vi "everything.vi"() -> ()   [LabVIEW 2019]
uses:
  <vilib>/Instr/_visa.llb/VISA Set IO Buffer Mask.ctl
  <vilib>/Instr/_visa.llb/VISA Configure Serial Port (Instr).vi
  <vilib>/express/express shared/transition.llb/Dynamic To Waveform Array.vi
  <vilib>/express/express arith-compare/Formula/Block/exnFormulaBlock how many pts in the wave.vi
  <vilib>/express/express shared/ex_Modify Signal Name.vi
  <vilib>/express/express shared/transition.llb/Waveform Array To Dynamic.vi
  <vilib>/express/express arith-compare/Formula/XNode/ExpressFormulaBlockNode.xnode
panel:
  out "VI Name":string
  out "Voltage 3":dbl format="%.2g"
  out "CFM 3":dbl format="%.2g"
  out "Average CFM 3":dbl format="%.1g"
  out "Voltage 2":dbl format="%#.2g"
  out "CFM 2":dbl format="%.2g"
  out "Average CFM 2":dbl format="%.1g"
  out "CFM 1":dbl format="%.2g"
  out "Average CFM 1":dbl format="%.1g"
  out "Voltage 1":dbl format="%#.2g"
  in  "% Power":dbl min=0.0 max=100.0 step=1.0
  out "Required Voltage":dbl
  out "main return":dbl
  out "t4":dbl
  out "zone 2":dbl
  out "t3":dbl
  out "outlet":dbl
  out "t6":dbl
  out "zone 1":dbl
  out "t5":dbl
  out "t2":dbl
  out "h2":dbl
  out "t1":dbl
  out "h3":dbl
  out "inlet air":dbl
  out "h4":dbl
  out "h1":dbl
  out "h6":dbl
  out "zone 3":dbl
  out "h5":dbl
  in  "Stop":bool
  in  "zone 1 inlet":dbl min=0.0 max=100.0
  in  "zone 1 return":dbl min=0.0 max=100.0
  in  "Fans":i32 min=0 max=1
  in  "zone 2 inlet":dbl min=0.0 max=100.0
  in  "zone 3 inlet":dbl min=0.0 max=100.0
  in  "zone 2 return":dbl min=0.0 max=100.0
  in  "zone 1 co2":dbl min=0.0 max=100.0
  in  "Light 1":i32 min=0 max=1
  in  "fresh air":dbl min=0.0 max=100.0
  in  "zone 2 co2":dbl min=0.0 max=100.0
  in  "Light 3":i32 min=0 max=1
  in  "zone 3 return":dbl min=0.0 max=100.0
  in  "Light 2":i32 min=0 max=1
  in  "zone 3 co2":dbl min=0.0 max=100.0
  in  "VISA- Arduino Uno":refnum<visa-resource-name>
  in  "VISA- Arduino Mega":refnum<visa-resource-name>
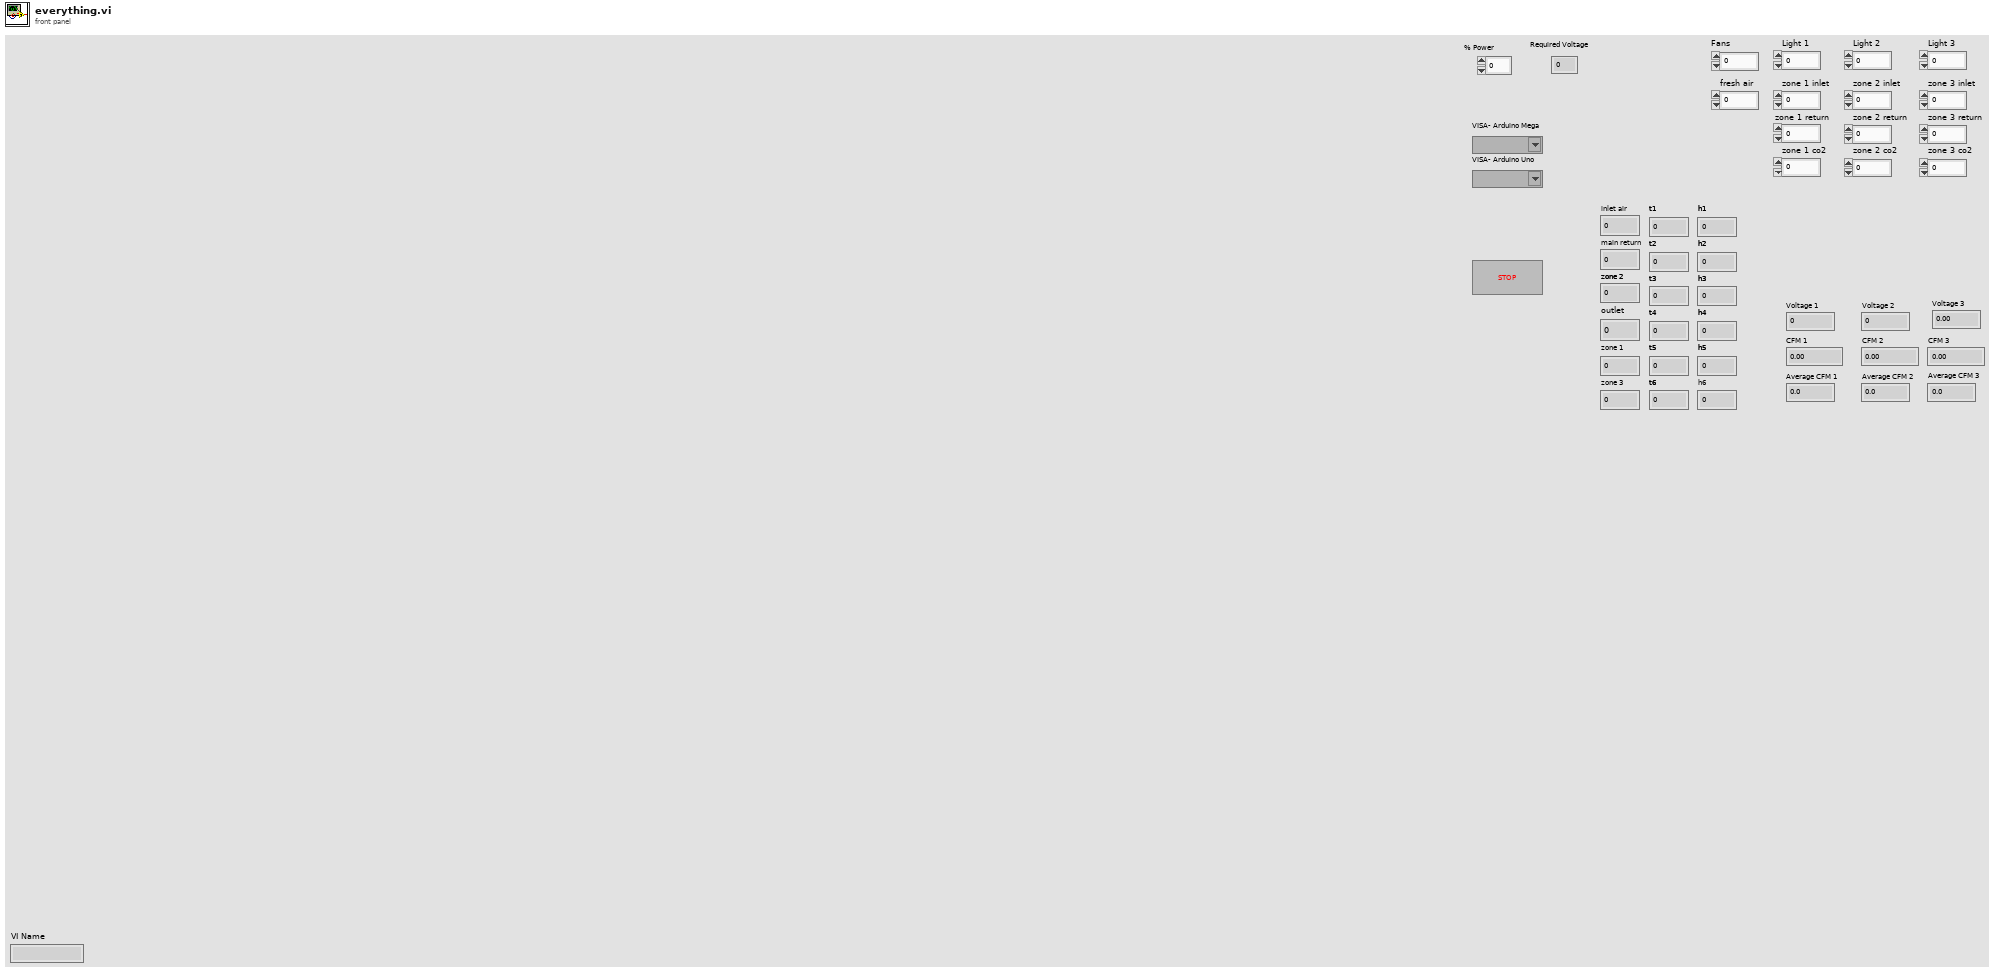
[diagram p1: front panel]
types:
  T1 = typedef "VISA Set IO Buffer Mask.ctl" = u16
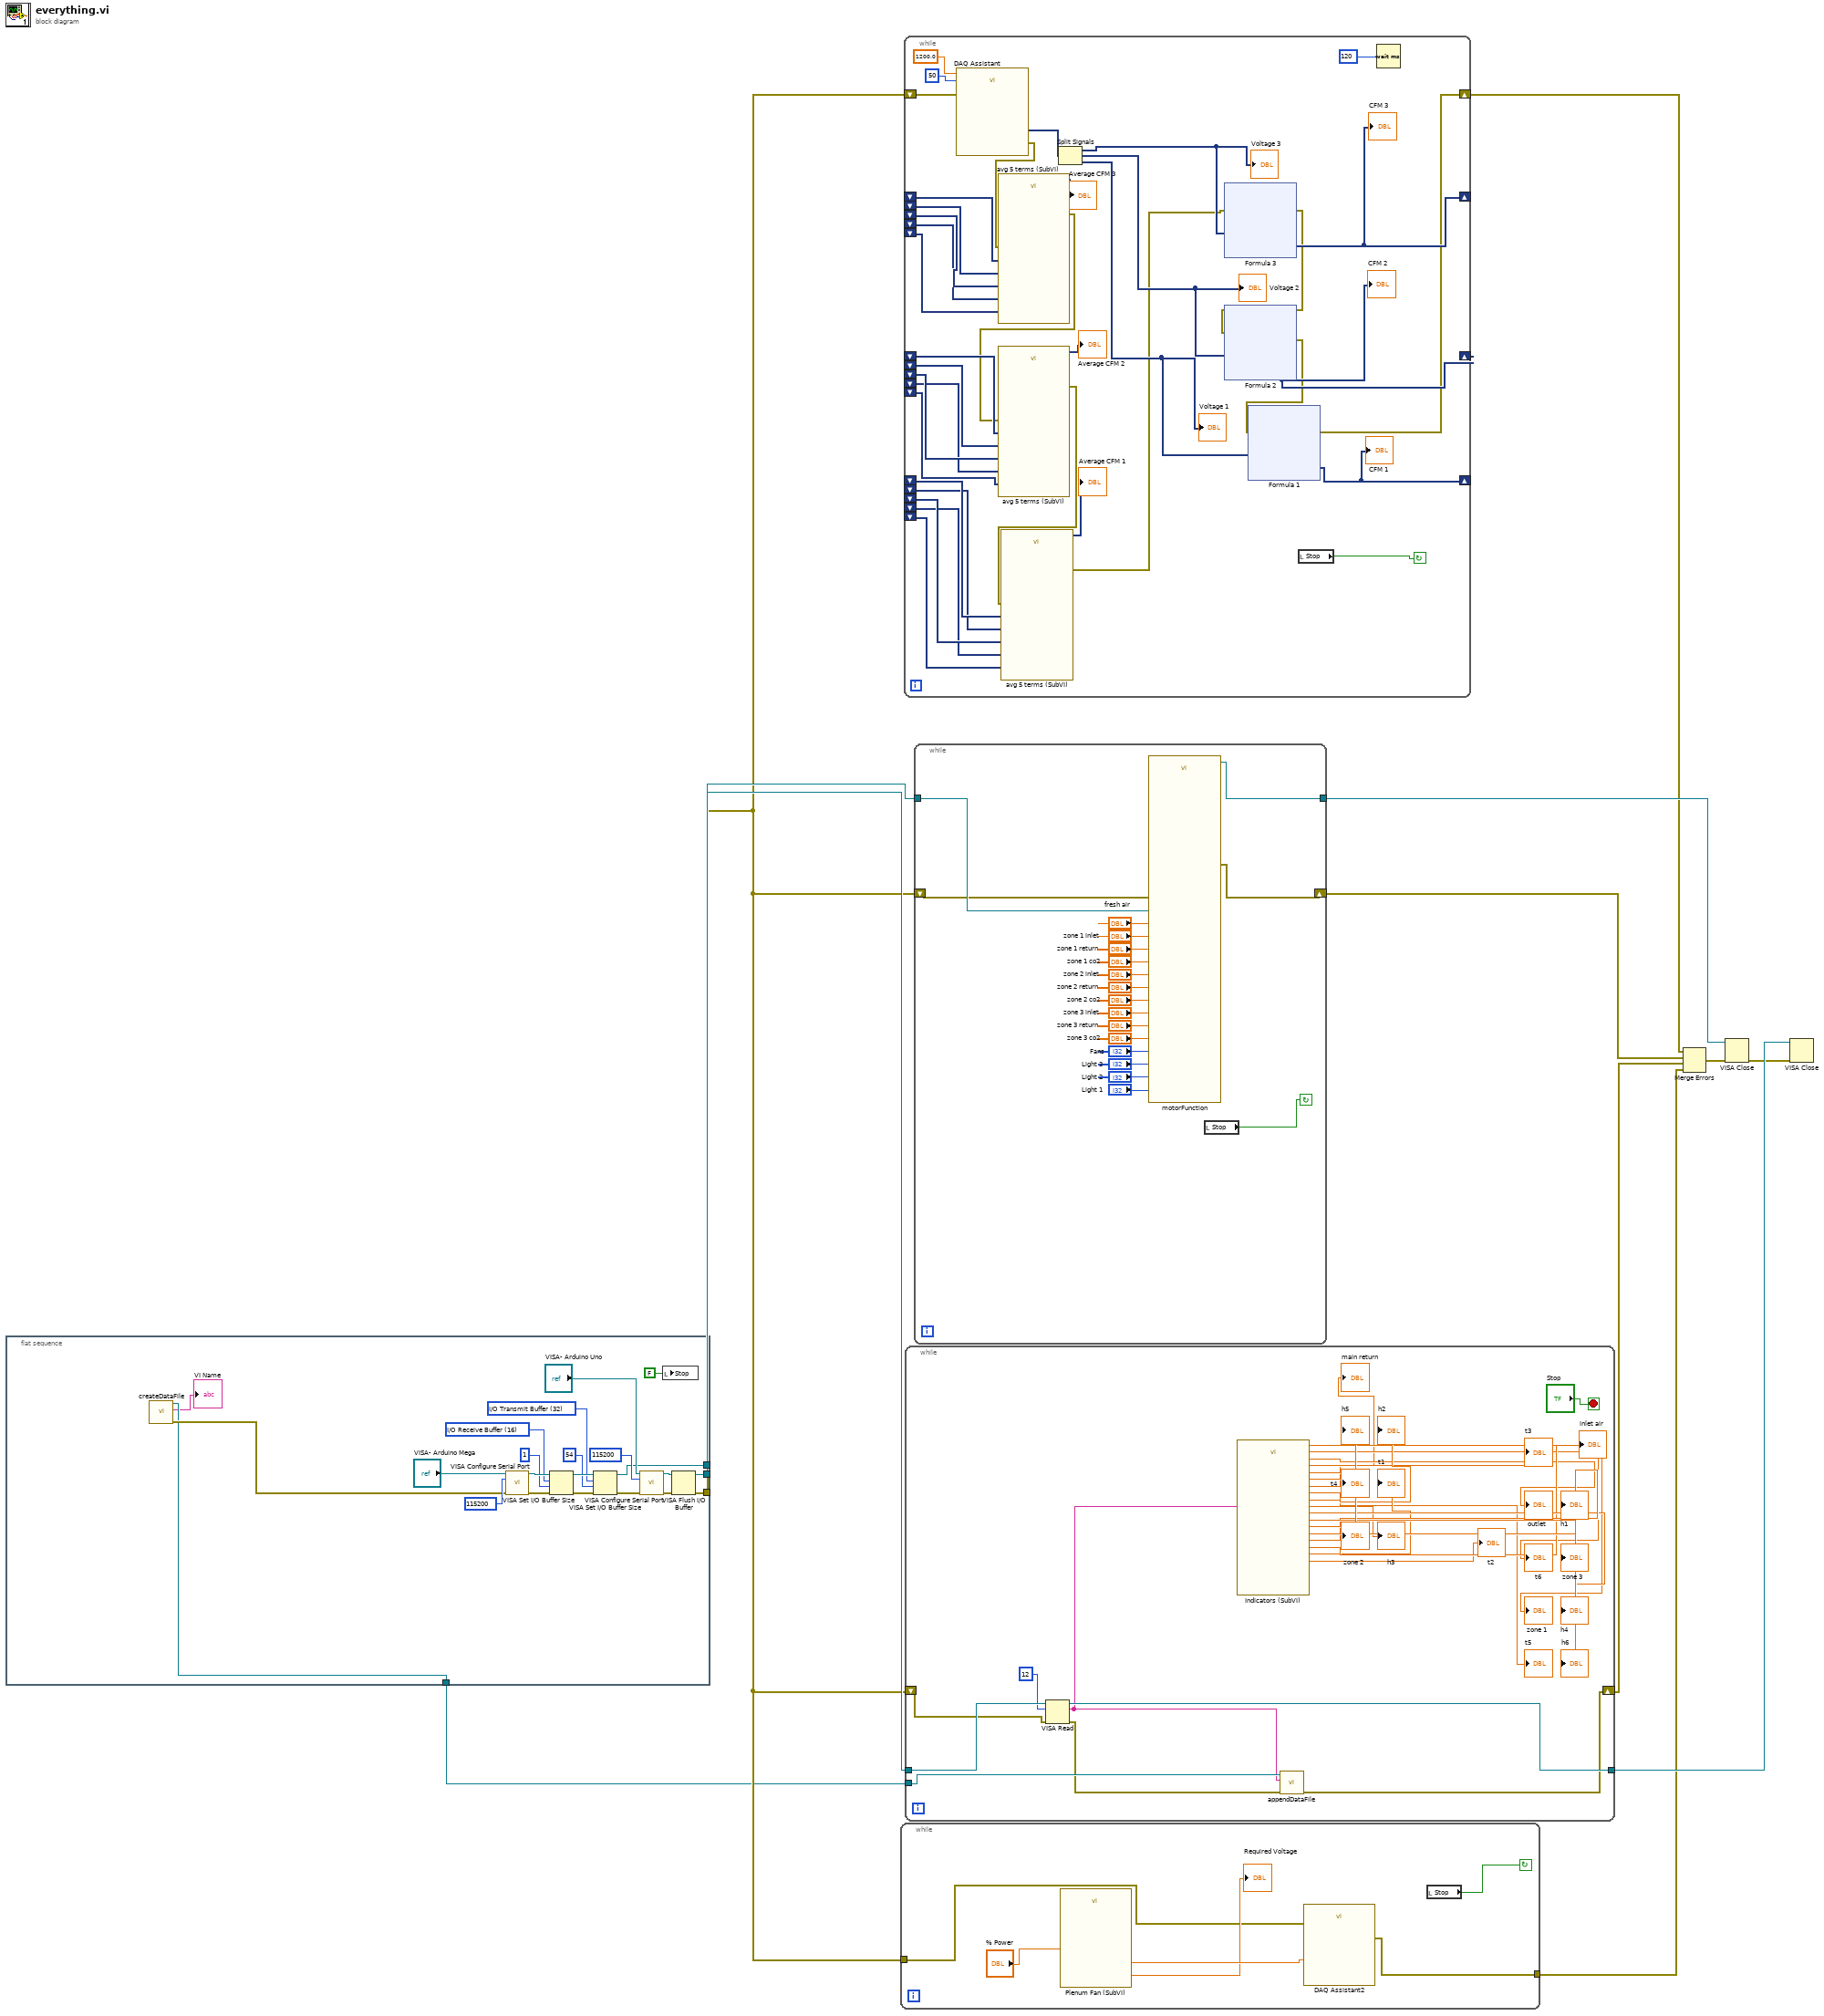
[diagram p0: block diagram]
diagram:
  n1 = flat-sequence {
    tunnel: [w20] -> w12
    tunnel: [w19] -> w11
    tunnel: [w17] -> w3
    tunnel: [w14] -> w1
    frame #0 {
      w27 = T1 32 items=["I/O Receive Buffer"=16, "I/O Transmit Buffer"=32, "I/O Receive and Transmit Buffer"=48] ("Mask")
      w30 = T1 16 items=["I/O Receive Buffer"=16, "I/O Transmit Buffer"=32, "I/O Receive and Transmit Buffer"=48] ("Mask")
      n2 = call "createDataFile.vi"() -> ("error out"=w15:errorcluster, "VI Name"=→"VI Name":string, "Byte Stream File out"=w14:refnum<file>)  [unwired: 9 in]
      n3 = call-poly "VISA Configure Serial Port"("VISA resource name"="VISA- Arduino Mega", "baud rate (115200)"=u32 115200 ("baud rate (9600)"), "error in (no error)"=w15) -> ("VISA resource name out"=w33:refnum<visa-resource-name>, "error out"=w32:errorcluster)  [unwired: 11 in]
      n4 = VISA Set I/O Buffer Size(VISA resource name=w33, mask (16)=w30, size (4096)=u32 1, error in (no error)=w32) -> (VISA resource name out=w28:refnum<visa-resource-name>, error out=w29:errorcluster)
      n5 = VISA Set I/O Buffer Size(VISA resource name=w28, mask (16)=w27, size (4096)=u32 54, error in (no error)=w29) -> (VISA resource name out=w19:refnum<visa-resource-name>, error out=w18:errorcluster)
      n6 = call-poly "VISA Configure Serial Port"("VISA resource name"="VISA- Arduino Uno", "baud rate (115200)"=u32 115200, "error in (no error)"=w18) -> ("VISA resource name out"=w22:refnum<visa-resource-name>, "error out"=w23:errorcluster)  [unwired: 11 in]
      n7 = local write "Stop"(FALSE ("Stop")) -> ()
      n8 = VISA Flush I/O Buffer(VISA resource name=w22, error in (no error)=w23) -> (VISA resource name out=w20:refnum<visa-resource-name>, error out=w17:errorcluster)  [unwired: 1 in]
    }
  }
  n9 = while {
    tunnel: [w37] -> w4
    tunnel: w3 -> [w36]
    stop <- w35 continue-if-true
    n10 = call "Plenum Fan (SubVI).vi"("% Power"="% Power") -> ("Numeric"=w39:dbl, "Required Voltage"=→"Required Voltage":dbl)  [unwired: 9 in]
    n11 = call "DAQ Assistant2"("data"=w39, "error in"=w36) -> ("error out"=w37:errorcluster)  [unwired: 16 in, 1 out]
    n12 = local read "Stop"() -> (w35:bool)
  }
  n13 = while {
    shift-right: [w72] -> _
    shift-left: _ -> [w53]
    shift-left: _ -> [w50]
    shift-left: _ -> [w51]
    shift-right: [w75] -> _
    shift-left: _ -> [w58]
    shift-left: _ -> [w56]
    shift-left: _ -> [w55]
    shift-left: _ -> [w52]
    shift-left: _ -> [w49]
    shift-left: _ -> [w57]
    shift-left: _ -> [w54]
    shift-right: [w74] -> _
    shift-left: _ -> [w63]
    shift-left: _ -> [w62]
    shift-left: _ -> [w61]
    shift-left: _ -> [w60]
    shift-left: _ -> [w59]
    shift-right: [w67] -> w2
    shift-left: w3 -> [w66]
    stop <- w41 continue-if-true
    n14 = call "DAQ Assistant"("rate"=1200.0, "number of samples"=50, "error in"=w66) -> ("data"=w77:dynamicdata, "error out"=w45:errorcluster)  [unwired: 14 in, 1 out]
    n15 = call "avg 5 terms (SubVI).vi"("Result"=w53, "Result 3"=w51, "error in (no error)"=w45, "Result 4"=w50, "Result 5"=w49, "Result 2"=w52) -> ("error out"=w44:errorcluster, "Dynamic Data"=→"Average CFM 3":dynamicdata)  [unwired: 4 in]
    n16 = call "avg 5 terms (SubVI).vi"("Result"=w58, "Result 3"=w56, "error in (no error)"=w44, "Result 4"=w55, "Result 5"=w54, "Result 2"=w57) -> ("error out"=w43:errorcluster, "Dynamic Data"=→"Average CFM 2":dynamicdata)  [unwired: 4 in]
    n17 = call "avg 5 terms (SubVI).vi"("Result"=w63, "Result 3"=w61, "error in (no error)"=w43, "Result 4"=w60, "Result 5"=w59, "Result 2"=w62) -> ("error out"=w42:errorcluster, "Dynamic Data"=→"Average CFM 1":dynamicdata)  [unwired: 4 in]
    n18 = Split Signals(w77) -> (w70:dynamicdata, w71:dynamicdata, w73:dynamicdata)  [unwired: 3 in]
    "Voltage 3" <- w70
    "Voltage 2" <- w71
    "Voltage 1" <- w73
    n19 = xnode "Formula 3"("X1"=w70, "error in (no error)"=w42) -> ("Result"=w72:dynamicdata, "error out"=w69:errorcluster)
    "CFM 3" <- w72
    n20 = xnode "Formula 2"("X1"=w71, "error in (no error)"=w69) -> ("Result"=w75:dynamicdata, "error out"=w68:errorcluster)
    "CFM 2" <- w75
    n21 = xnode "Formula 1"("X1"=w73, "error in (no error)"=w68) -> ("Result"=w74:dynamicdata, "error out"=w67:errorcluster)
    "CFM 1" <- w74
    n22 = local read "Stop"() -> (w41:bool)
    n23 = Wait (ms)(milliseconds to wait=u32 120 ("millisecond timer value")) -> ()  [unwired: 1 out]
  }
  n24 = while {
    shift-right: [w497] -> w6
    shift-left: w3 -> [w519]
    tunnel: w12 -> [w521]
    tunnel: [w520] -> w10
    tunnel: w1 -> [w499]
    stop <- "Stop" stop-if-true
    n25 = VISA Read(VISA resource name=w521, byte count=u32 12, error in (no error)=w519) -> (VISA resource name out=w520:refnum<visa-resource-name>, read buffer=w496:string, error out=w498:errorcluster)  [unwired: 1 out]
    n26 = call "Indicators (SubVI).vi"("read buffer"=w496) -> ("h5"=→"h5":dbl, "zone 3"=→"zone 3":dbl, "h6"=→"h6":dbl, "h1"=→"h1":dbl, "h4"=→"h4":dbl, "inlet air"=→"inlet air":dbl, "h3"=→"h3":dbl, "t1"=→"t1":dbl, "h2"=→"h2":dbl, "t2"=→"t2":dbl, "t5"=→"t5":dbl, "zone 1"=→"zone 1":dbl, "t6"=→"t6":dbl, "outlet"=→"outlet":dbl, "t3"=→"t3":dbl, "zone 2"=→"zone 2":dbl, "t4"=→"t4":dbl, "main return"=→"main return":dbl)  [unwired: 9 in]
    n27 = call "appendDataFile.vi"("error in (no error)"=w498, "read buffer"=w496, "Byte Stream File in"=w499) -> ("error out"=w497:errorcluster)  [unwired: 8 in]
  }
  n28 = while {
    shift-right: [w524] -> w7
    shift-left: w3 -> [w526]
    tunnel: w11 -> [w527]
    tunnel: [w525] -> w5
    stop <- w522 continue-if-true
    n29 = call "motorFunction.vi"("VISA Refnum in"=w527, "zone 3 co2"="zone 3 co2", "Light 2"="Light 2", "zone 3 return"="zone 3 return", "Light 1"="Light 3", "zone 2 co2"="zone 2 co2", "fresh air"="fresh air", "error in (no error)"=w526, "Light 3"="Light 1", "zone 1 co2"="zone 1 co2", "zone 2 return"="zone 2 return", "zone 3 inlet"="zone 3 inlet", "zone 2 inlet"="zone 2 inlet", "Fans"="Fans", "zone 1 return"="zone 1 return", "zone 1 inlet"="zone 1 inlet") -> ("VISA Refnum out"=w525:refnum<visa-resource-name>, "error out"=w524:errorcluster)  [unwired: 10 in]
    n30 = local read "Stop"() -> (w522:bool)
  }
  n31 = Merge Errors(w2, w7, w6, w4) -> (w8:errorcluster)
  n32 = VISA Close(VISA resource name=w5, error in (no error)=w8) -> (error out=w9:errorcluster)
  n33 = VISA Close(VISA resource name=w10, error in (no error)=w9) -> ()  [unwired: 1 out]
